vi "nanocal -- nuclear schottky fit -- 2x2 -- V9.vi"() -> ()   [LabVIEW 2021] (continued)
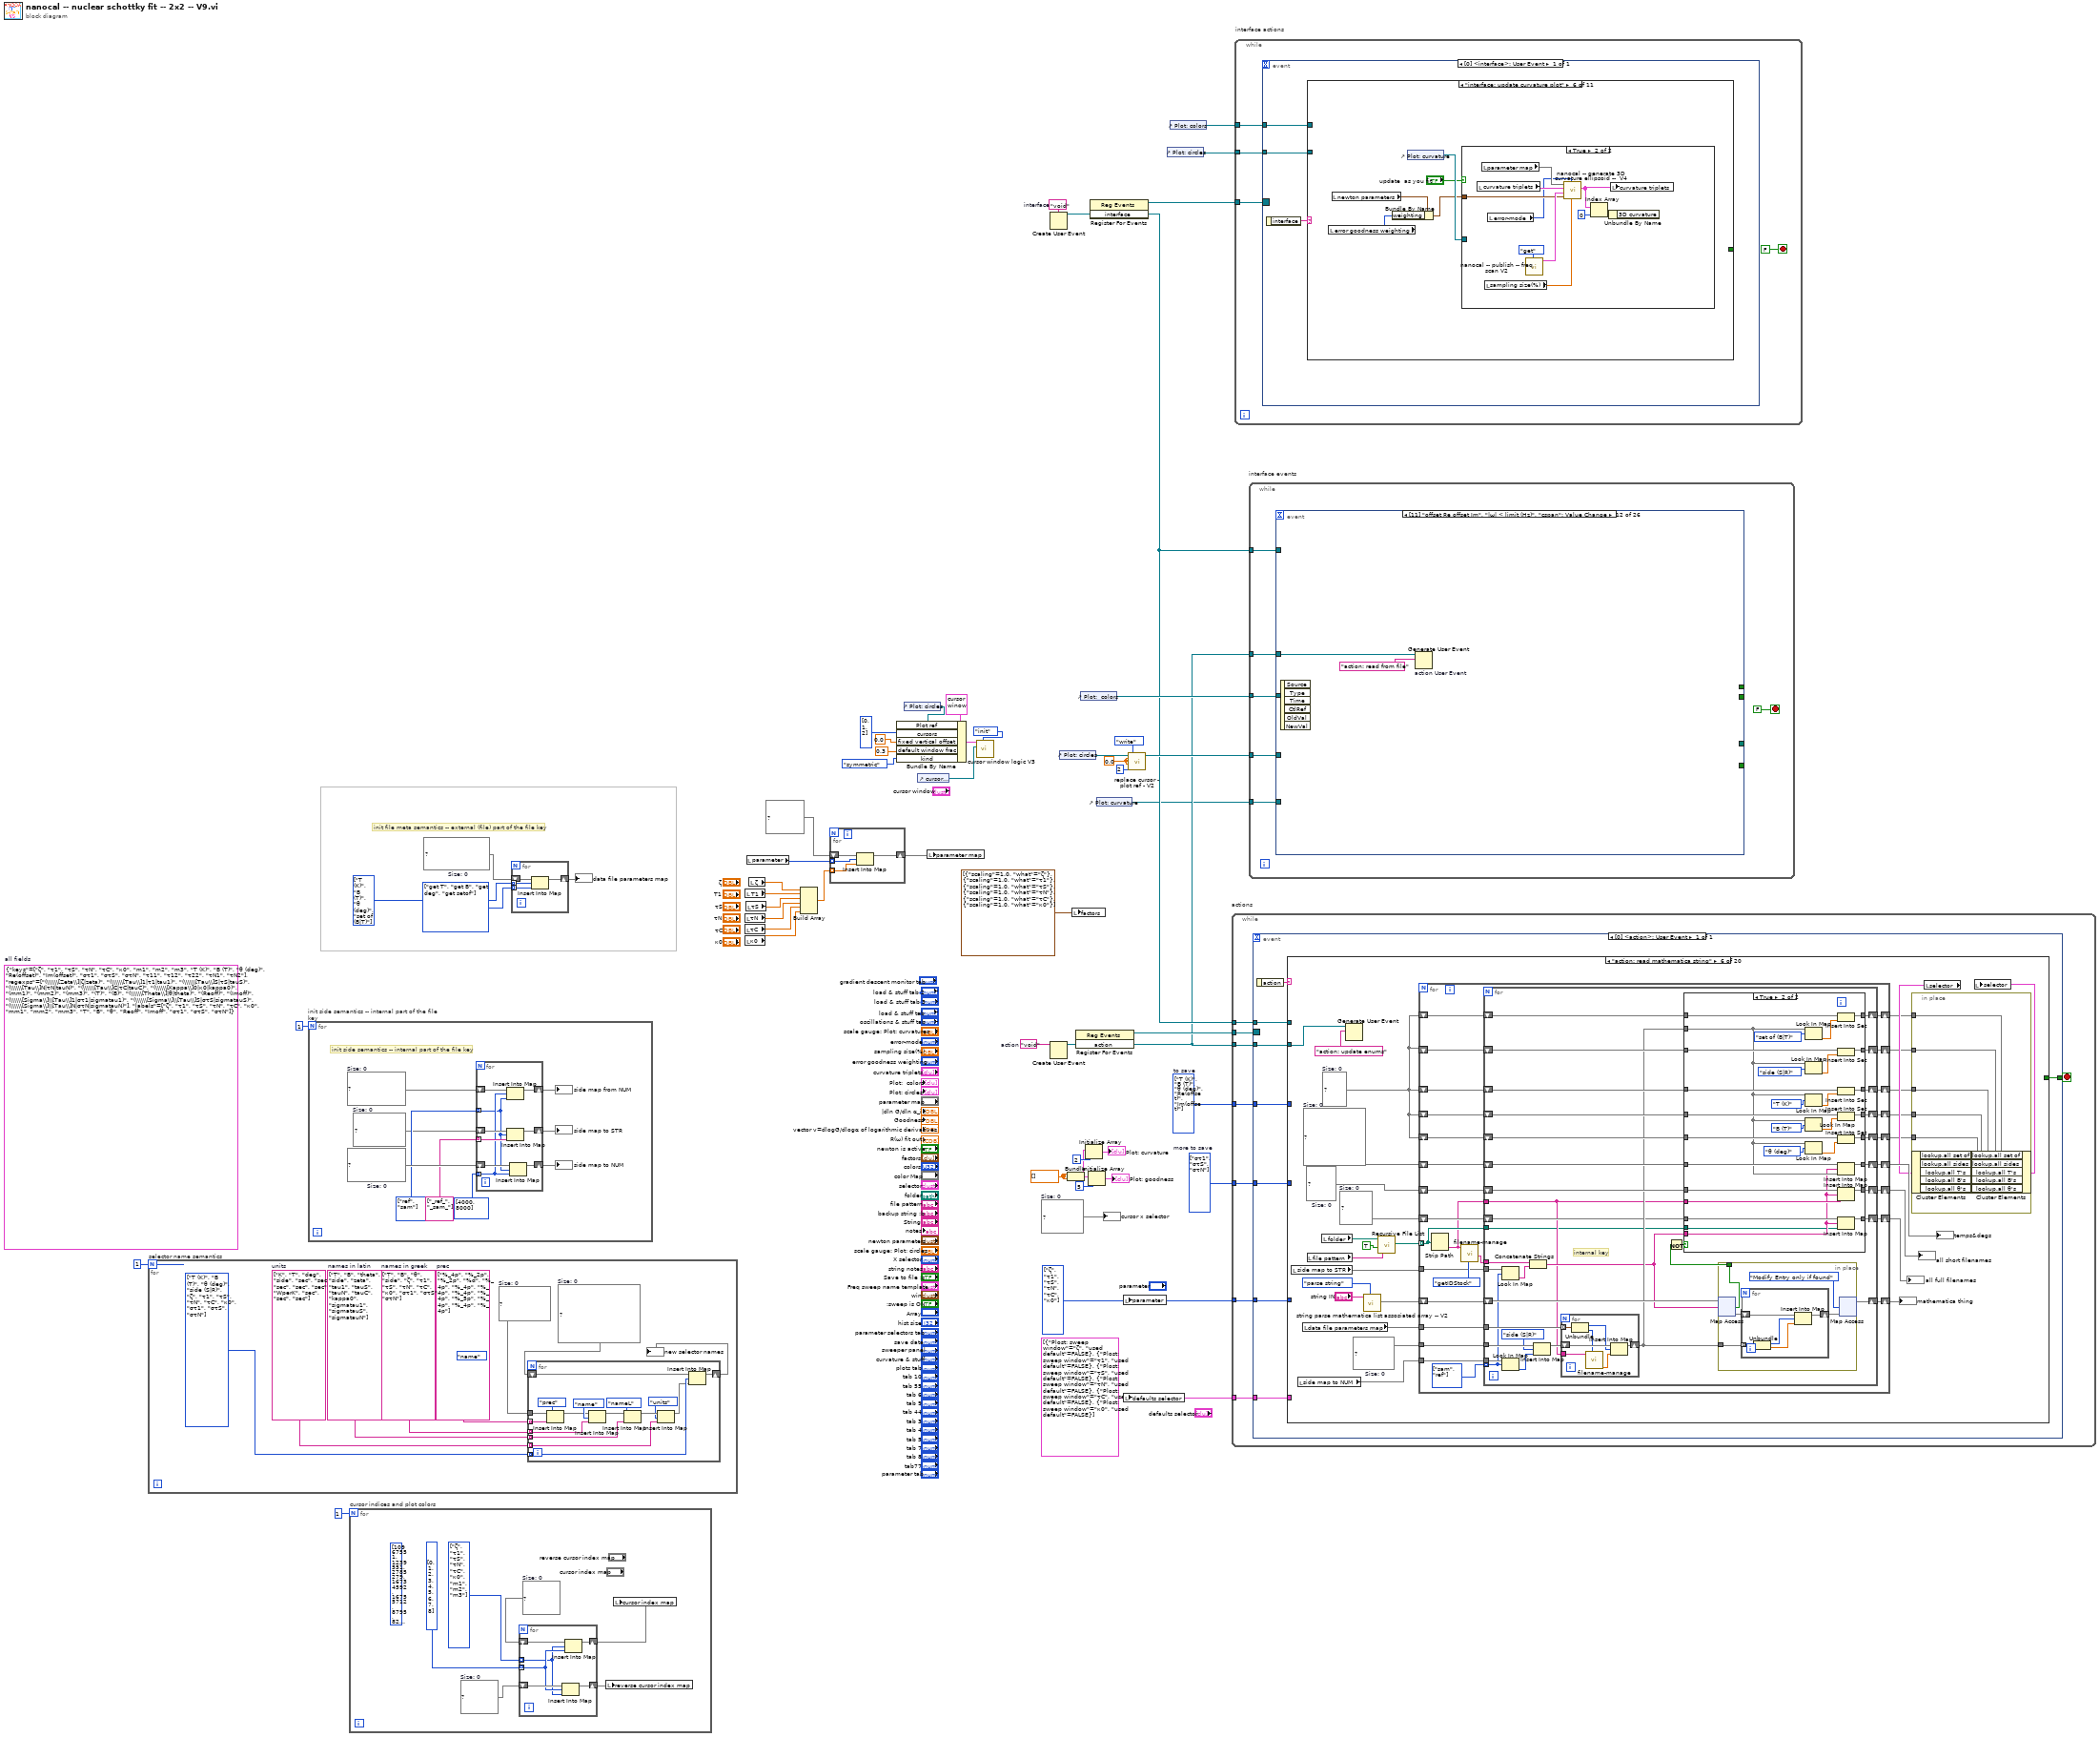
[diagram p0: block diagram]
diagram:
  w1 = T2[] [enum."T (K)", enum."B (T)", enum."θ (deg)", enum."Re(offset)", enum."Im(offset)"] items=["ζ", "τ1", "τS", "τN", "τC", "κ0", "m1", "m2", "m3", "T (K)", "B (T)", "θ (deg)", "side (S|R)", "set of (B|T)", "Re(offset)", "Im(offset)", "στ1", "στ1-", "στ1+", "στS", "στS-", "στS+", "στN", "στN-", "στN+", "τ11", "τ12", "τ21", "τ22", "τN1", "τN2"]  # to save
  w2 = T2[] [enum."στ1", enum."στS", enum."στN"] items=["ζ", "τ1", "τS", "τN", "τC", "κ0", "m1", "m2", "m3", "T (K)", "B (T)", "θ (deg)", "side (S|R)", "set of (B|T)", "Re(offset)", "Im(offset)", "στ1", "στ1-", "στ1+", "στS", "στS-", "στS+", "στN", "στN-", "στN+", "τ11", "τ12", "τ21", "τ22", "τN1", "τN2"]  # more to save
  (unwired) T20 {"keys"=[enum."ζ", enum."τ1", enum."τS", enum."τN", enum."τC", enum."κ0", enum."m1", enum."m2", enum."m3", enum."T (K)", enum."B (T)", enum."θ (deg)", enum."Re(offset)", enum."Im(offset)", enum."στ1", enum."στS", enum."στN", enum."τ11", enum."τ12", enum."τ22", enum."τN1", enum."τN2"], "regexps"=["(\\\\\\[Zeta\\]|ζ|zeta)", "(\\\\\\[Tau\\]1|τ1|tau1)", "(\\\\\\[Tau\\]S|τS|tauS)", "(\\\\\\[Tau\\]N|τN|tauN)", "(\\\\\\[Tau\\]C|τC|tauC)", "(\\\\\\[Kappa\\]0|κ0|kappa0)", "(mm1)", "(mm2)", "(mm3)", "(T)", "(B)", "(\\\\\\[Theta\\]|θ|theta)", "(Reoff)", "(Imoff)", "(\\\\\\[Sigma\\]\\[Tau\\]1|στ1|sigmatau1)", "(\\\\\\[Sigma\\]\\[Tau\\]S|στS|sigmatauS)", "(\\\\\\[Sigma\\]\\[Tau\\]N|στN|sigmatauN)"], "labels"=["ζ", "τ1", "τS", "τN", "τC", "κ0", "mm1", "mm2", "mm3", "T", "B", "θ", "Reoff", "Imoff", "στ1", "στS", "στN"]}  # all fields
  w26 = T9 [{"Plost: sweep window"=enum."ζ", "used default"=FALSE}, {"Plost: sweep window"=enum."τ1", "used default"=FALSE}, {"Plost: sweep window"=enum."τS", "used default"=FALSE}, {"Plost: sweep window"=enum."τN", "used default"=FALSE}, {"Plost: sweep window"=enum."τC", "used default"=FALSE}, {"Plost: sweep window"=enum."κ0", "used default"=FALSE}] ("parameter 2")
  w27 = T18[] [enum."get T", enum."get B", enum."get deg", enum."get setof"] items=["rewrite", "parse", "force pattern", "uniquenum", "get T", "get B", "get ind", "get deg", "get name", "get folder", "get extension", "get basename", "get side", "get setof", "getID", "getIDStock"]
  w29 = map{T2, T18} {}  # Size: 0
  w28 = T2[] [enum."T (K)", enum."B (T)", enum."θ (deg)", enum."set of (B|T)"] items=["ζ", "τ1", "τS", "τN", "τC", "κ0", "m1", "m2", "m3", "T (K)", "B (T)", "θ (deg)", "side (S|R)", "set of (B|T)", "Re(offset)", "Im(offset)", "στ1", "στ1-", "στ1+", "στS", "στS-", "στS+", "στN", "στN-", "στN+", "τ11", "τ12", "τ21", "τ22", "τN1", "τN2"]
  w33 = dbl[] []
  w22 = T2[] [enum."ζ", enum."τ1", enum."τS", enum."τN", enum."τC", enum."κ0"] items=["ζ", "τ1", "τS", "τN", "τC", "κ0", "m1", "m2", "m3", "T (K)", "B (T)", "θ (deg)", "side (S|R)", "set of (B|T)", "Re(offset)", "Im(offset)", "στ1", "στ1-", "στ1+", "στS", "στS-", "στS+", "στN", "στN-", "στN+", "τ11", "τ12", "τ21", "τ22", "τN1", "τN2"]
  w36 = map{T2, dbl} {}  # Size: 0
  w37 = 0.0 ("new X")
  w50 = "void"  # interface
  w51 = "void"  # action
  # "init file meta semantics -- external (file) part of the file key"
  n1 = for "selector name semantics" {
    N: 1 -> [_]
    w53 = string[] ["%_4p", "%_2p", "%_2p", "%d", "%_4p", "%_4p", "%_4p", "%_4p", "%_4p", "%_5p", "%_4p", "%_4p", "%_4p"]  # prec
    w57 = map{T19, string} {}  # Size: 0
    (unwired) nameformattingitem."name" ("name formatting item")
    w55 = string[] ["K", "T", "deg", "side", "sec", "sec", "sec", "sec", "sec", "WperK", "sec", "sec", "sec"]  # units
    w58 = string[] ["T", "B", "theta", "side", "zeta", "tau1", "tauS", "tauN", "tauC", "kappa0", "sigmatau1", "sigmatauS", "sigmatauN"]  # names in latin
    w56 = string[] ["T", "B", "θ", "side", "ζ", "τ1", "τS", "τN", "τC", "κ0", "στ1", "στS", "στN"]  # names in greek
    w60 = map{T2, map{T19, string}} {}  # Size: 0
    w59 = T2[] [enum."T (K)", enum."B (T)", enum."θ (deg)", enum."side (S|R)", enum."ζ", enum."τ1", enum."τS", enum."τN", enum."τC", enum."κ0", enum."στ1", enum."στS", enum."στN"] items=["ζ", "τ1", "τS", "τN", "τC", "κ0", "m1", "m2", "m3", "T (K)", "B (T)", "θ (deg)", "side (S|R)", "set of (B|T)", "Re(offset)", "Im(offset)", "στ1", "στ1-", "στ1+", "στS", "στS-", "στS+", "στN", "στN-", "στN+", "τ11", "τ12", "τ21", "τ22", "τN1", "τN2"]
    n2 = for {
      shift-right: [w75] -> w54
      shift-left: w60 -> [w76]
      tunnel: w58 -> [w66] mode=indexing
      tunnel: w59 -> [w74] mode=indexing
      tunnel: w57 -> [w64]
      tunnel: w56 -> [w65] mode=indexing
      tunnel: w55 -> [w67] mode=indexing
      tunnel: w53 -> [w63] mode=indexing
      n3 = Insert Into Map(map in=w64, key=nameformattingitem."prec", value=w63) -> (map out=w62:map{T19, string})  [unwired: 2 out]
      n4 = Insert Into Map(map in=w62, key=nameformattingitem."name", value=w65) -> (map out=w73:map{T19, string})  [unwired: 2 out]
      n5 = Insert Into Map(map in=w73, key=nameformattingitem."nameL" ("name formatting item"), value=w66) -> (map out=w72:map{T19, string})  [unwired: 2 out]
      n6 = Insert Into Map(map in=w72, key=nameformattingitem."units" ("name formatting item"), value=w67) -> (map out=w71:map{T19, string})  [unwired: 2 out]
      n7 = Insert Into Map(map in=w76, key=w74, value=w71) -> (map out=w75:map{T2, map{T19, string}})  [unwired: 2 out]
    }
    "new selector names" <- w54
  }
  n8 = for "init side semantics -- internal part of the file key" {
    N: 1 -> [_]
    w78 = map{i32, T8} {}  # Size: 0
    w80 = map{T8, string} {}  # Size: 0
    w81 = T8[] [enum."ref", enum."sam"] items=["sam", "ref"]
    w85 = map{T8, i32} {}  # Size: 0
    # "init side semantics -- internal part of the file key"
    n9 = for {
      shift-right: [w93] -> w82
      shift-left: w85 -> [w94]
      tunnel: string[] ["_ref_", "_sam_"] -> [w90] mode=indexing
      tunnel: i32[] [4000, 8000] -> [w87] mode=indexing
      tunnel: w81 -> [w86] mode=indexing
      shift-right: [w91] -> w79
      shift-left: w80 -> [w92]
      shift-right: [w88] -> w77
      shift-left: w78 -> [w89]
      n10 = Insert Into Map(map in=w89, key=w87, value=w86) -> (map out=w88:map{i32, T8})  [unwired: 2 out]
      n11 = Insert Into Map(map in=w92, key=w86, value=w90) -> (map out=w91:map{T8, string})  [unwired: 2 out]
      n12 = Insert Into Map(map in=w94, key=w86, value=w87) -> (map out=w93:map{T8, i32})  [unwired: 2 out]
    }
    "side map from NUM" <- w77
    "side map to STR" <- w79
    "side map to NUM" <- w82
  }
  n13 = for "cursor indices and plot colors" {
    N: 1 -> [_]
    w96 = map{i32, T2} {}  # Size: 0
    (unwired) u32[] [10967551, 1239551, 2785279, 16734592, 16755712, 8795, 8285330, 9272482, 9204890]
    w100 = map{T2, i32} {}  # Size: 0
    w97 = T2[] [enum."ζ", enum."τ1", enum."τS", enum."τN", enum."τC", enum."κ0", enum."m1", enum."m2", enum."m3"] items=["ζ", "τ1", "τS", "τN", "τC", "κ0", "m1", "m2", "m3", "T (K)", "B (T)", "θ (deg)", "side (S|R)", "set of (B|T)", "Re(offset)", "Im(offset)", "στ1", "στ1-", "στ1+", "στS", "στS-", "στS+", "στN", "στN-", "στN+", "τ11", "τ12", "τ21", "τ22", "τN1", "τN2"]
    n14 = for {
      shift-right: [w105] -> w98
      shift-left: w100 -> [w106]
      tunnel: w97 -> [w101] mode=indexing
      tunnel: i32[] [0, 1, 2, 3, 4, 5, 6, 7, 8] -> [w102] mode=indexing
      shift-right: [w103] -> w95
      shift-left: w96 -> [w104]
      n15 = Insert Into Map(map in=w104, key=w102, value=w101) -> (map out=w103:map{i32, T2})  [unwired: 2 out]
      n16 = Insert Into Map(map in=w106, key=w101, value=w102) -> (map out=w105:map{T2, i32})  [unwired: 2 out]
    }
    n17 = local write "reverse cursor index map"(w95) -> ()
    n18 = local write "cursor index map"(w98) -> ()
  }
  n19 = for {
    shift-right: [w109] -> w30
    shift-left: w29 -> [w110]
    tunnel: w28 -> [w108] mode=indexing
    tunnel: w27 -> [w107] mode=indexing
    n20 = Insert Into Map(map in=w110, key=w108, value=w107) -> (map out=w109:map{T2, T18})  [unwired: 2 out]
  }
  "data file parameters map" <- w30
  n21 = local read "τN"() -> (w16:dbl)
  n22 = local read "τC"() -> (w17:dbl)
  n23 = local read "κ0"() -> (w18:dbl)
  n24 = local read "T1"() -> (w14:dbl)
  n25 = local read "τS"() -> (w15:dbl)
  n26 = local read "parameter"() -> (w20:T2[])
  n27 = local read "ζ"() -> (w13:dbl)
  n28 = Build Array(w13, w14, w15, w16, w17, w18) -> (w19:dbl[])
  n29 = for {
    shift-right: [w113] -> w21
    shift-left: map{T2, dbl} {} ("Map IN") -> [w114]
    tunnel: w20 -> [w112] mode=indexing
    tunnel: w19 -> [w111] mode=indexing
    n30 = Insert Into Map(map in=w114, key=w112, value=w111) -> (map out=w113:map{T2, dbl})  [unwired: 2 out]
  }
  n31 = control-ref of="Plot: circles"() -> (w42:refnum<vi>)
  n32 = Bundle By Name(cluster=T17 {"left"=0.0, "right "=0.0, "center"=0.0, "window"=0.0, "cursors"=[], "relative"=0, "absolute"=0, "fixed vertical offset"=0.0, "vertical offset"=0.0, "skew"=0.0, "default window frac"=0.0, "kind"=enum."symmetric", "skew.left"=0.0, "skew.right"=0.0, "Plot ref"=refnum, "wing order"=enum."forw"} ("cursor bracket: All, data window"), "Plot ref"=w42, "cursors"=i32[] [0, 1, 2], "fixed vertical offset"=0.0, "default window frac"=0.3 ("fixed vertical offset"), "kind"=enum16{"symmetric", "skewed", "fancy"}."symmetric") -> (w45:T17)
  n33 = control-ref of="cursor window"() -> (w41:refnum<vi>)
  n34 = local write "parameter map"(w21) -> ()
  n35 = call "cursor window logic V3.vi"("cursor window action"=cursor_window_action."init", "cursor window in"=w41, "cursor window init"=w45) -> ()  [unwired: 7 in, 2 out]
  n36 = Create User Event(user event datatype=w50) -> (user event=w10:refnum<user-event>)  [unwired: 1 in, 1 out]
  n37 = Create User Event(user event datatype=w51) -> (user event=w9:refnum<user-event>)  [unwired: 1 in, 1 out]
  n38 = control-ref of="Plot: circles"() -> (w38:refnum<vi>)
  n39 = Bundle(w33, w33) -> (w5:cluster{dbl[], dbl[]})  [unwired: 1 in]
  n40 = local write "factors"(cluster{"scaling":dbl, "what":T2}[] [{"scaling"=1.0, "what"=enum."ζ"}, {"scaling"=1.0, "what"=enum."τ1"}, {"scaling"=1.0, "what"=enum."τS"}, {"scaling"=1.0, "what"=enum."τN"}, {"scaling"=1.0, "what"=enum."τC"}, {"scaling"=1.0, "what"=enum."κ0"}]) -> ()
  n41 = register-events(w9) -> (reference out=w52:refnum<event-registration>)  [unwired: 2 in, 1 out]
  n42 = control-ref of="Plot:  colors"() -> (w35:refnum<vi>)
  n43 = Initialize Array(w5, 2 ("dimension size")) -> (→"Plot: curvature":cluster{dbl[], dbl[]}[])
  n44 = Initialize Array(w5, 5 ("dimension size")) -> (→"Plot: goodness":cluster{dbl[], dbl[]}[])
  n45 = register-events(w10) -> (reference out=w11:refnum<event-registration>)  [unwired: 2 in, 1 out]
  n46 = control-ref of="Plot: curvature"() -> (w3:refnum<vi>)
  n47 = local write "parameter"(w22) -> ()
  n48 = local write "defaults selector"(w26) -> ()
  n49 = call "replace cursor - plot ref - V2.vi"("Plot ref in"=w38, "new X"=w37, "new  Y"=w37, "cursor index"=2, "cursor action"=cursor_action."write") -> ()  [unwired: 11 in, 4 out]
  n50 = control-ref of="Plot: circles"() -> (w7:refnum<vi>)
  n51 = control-ref of="Plot: colors"() -> (w8:refnum<vi>)
  n52 = while "actions" {
    tunnel: w52 -> [w122]
    tunnel: w9 -> [w121]
    tunnel: w10 -> [w119]
    tunnel: w22 -> [w118]
    tunnel: w26 -> [w117]
    tunnel: w2 -> [w116]
    tunnel: w1 -> [w115]
    stop <- w120 stop-if-true
    n53 = event shown="[0] <action>: User Event" {
      selector: w122 -> [_]
      dyn-events: _ -> [_]
      timeout: _ -> [_]
      tunnel: w121 -> [w129]
      tunnel: [w128] -> w120
      tunnel: w119 -> [w127]
      tunnel: w118 -> [w126]
      tunnel: w117 -> [w125]
      tunnel: w116 -> [w124]
      tunnel: w115 -> [w123]
      event User Event {
        n54 = event-data() -> ("action"=w130:string)  [unwired: 1 in]
        n55 = case shown="\"action: read mathematica string\"" w130 {
          tunnel: w129 -> [w138 _ _ _ w321 w346 _ _ w539 _ w666 _ _ w772 w824 w925 _ w987 _ _]
          tunnel: [_ _ _ _ _ _ _ _ _ _ _ _ _ _ _ _ TRUE _ _ _] -> w128
          tunnel: w127 -> [w141 w145 _ w266 w315 _ _ _ _ _ _ _ w682 _ w814 _ _ _ _ _]
          tunnel: w126 -> [_ w152 w161 w265 _ _ w473 _ _ _ _ _ w680 _ w820 _ _ _ _ _]
          tunnel: w125 -> [_ _ _ _ _ _ _ _ _ _ _ _ _ _ _ _ _ _ _ _]
          tunnel: w124 -> [_ _ _ _ _ _ _ _ _ _ _ _ w678 _ _ w896 _ _ _ _]
          tunnel: w123 -> [_ _ _ _ _ _ _ _ _ _ _ _ _ _ _ w893 _ _ _ _]
          frame "action: new sweep" {
            n56 = Generate User Event(user event=w141, event data cluster="interface: update plot colors cursors" ("event data")) -> (user event out=w142:refnum<user-event>)  [unwired: 2 in, 1 out]
            n57 = Generate User Event(user event=w142, event data cluster="interface: reset colors" ("event data")) -> ()  [unwired: 2 in, 2 out]
            n58 = Generate User Event(user event=w138, event data cluster="action: replot circles" ("event data")) -> ()  [unwired: 2 in, 2 out]
            n59 = call "nanocal -- publish -- freq scan V2.vi"("publisher action"=publisher_action."get") -> ("z out (V)"=w137:cdb[])  [unwired: 7 in, 3 out]
            n60 = control-ref of="Plot: circles"() -> (w132:refnum<vi>)
            n61 = Complex To Re/Im(x + iy=w137) -> (x=w135:dbl[], y=w136:dbl[])
            n62 = call "replace plot - plot ref - V2.vi"("Plot ref in"=w132, "Array X IN"=w135, "Array Y IN"=w136, "plot index"=enum16{"data R(ω)", "fit R(ω)"}."data R(ω)" ("Plost: sweep window"), "cursor action"=cursor_action."write") -> ()  [unwired: 11 in, 4 out]
          }
          frame "action: replot circles" {
            n63 = local read "newton parameters"() -> (w153:T3)
            n64 = local read "parameter map"() -> (w147:map{T2, dbl})
            n65 = call "nanocal -- publish -- freq scan V2.vi"("publisher action"=publisher_action."get") -> ("data"=w151:T34)  [unwired: 7 in, 3 out]
            n66 = call "nanocal -- gradient descent.vi"("data"=w151, "action"=nanocal_--_gradient_descent_--_action."peek", "newton pars"=w153, "parameter keys IN"=w152, "parameter Map IN"=w147) -> ("logarithmic derivatives OUT"=w148:dbl[], "R(ω) out"=w146:cdb[], "goodness OUT"=w150:dbl)  [unwired: 2 in, 2 out]
            n67 = local write "vector v=dlogG/dlogα of logarithmic derivatives"(w148) -> ()
            n68 = Absolute Value(x=w148) -> (abs(x)=w149:dbl[])
            n69 = flat-sequence {
              tunnel: w146 -> [w156]
              tunnel: w145 -> [w158]
              tunnel: "interface: update circle fit plot" ("event data") -> [w157]
              frame #0 {
                n70 = local write "R(ω) fit out"(w156) -> ()
              }
              frame #1 {
                n71 = Generate User Event(user event=w158, event data cluster=w157) -> ()  [unwired: 2 in, 2 out]
              }
            }
            n72 = local write "Goodness"(w150) -> ()
            n73 = local write "|v_i| = | dlogG/dlogα_i | (log scale slider)"(w149) -> ()
          }
          frame "action: plot landscape" {
            w172 = array_action."generate log range" ("action")
            n74 = property on="range one" class="Slide (strict)"() -> ("Scale.Range"=w181:T36)  [unwired: 2 in, 2 out]
            n75 = property on="range two" class="Slide (strict)"() -> ("Scale.Range"=w180:T36)  [unwired: 2 in, 2 out]
            n76 = Unbundle By Name(w181) -> ("Maximum"=w175:dbl, "Minimum"=w174:dbl)
            n77 = Unbundle By Name(w180) -> ("Maximum"=w177:dbl, "Minimum"=w176:dbl)
            n78 = local read "cursor index map"() -> (w167:map{T2, i32})
            n79 = call "array -- generate range -- V5.vi"("action"=w172, "ω points"="# points", "ω from"=w176, "ω to"=w177) -> ("ω out"=w178:dbl[])  [unwired: 7 in]
            n80 = local read "color Map"() -> (w168:map{T2, u32})
            n81 = call "array -- generate range -- V5.vi"("action"=w172, "ω points"="# points", "ω from"=w174, "ω to"=w175) -> ("ω out"=w173:dbl[])  [unwired: 7 in]
            n82 = call "nanocal -- publish -- freq scan V2.vi"("publisher action"=publisher_action."get") -> ("data"=w160:T34)  [unwired: 7 in, 3 out]
            n83 = local read "newton parameters"() -> (w162:T3)
            n84 = local read "parameter map"() -> (w159:map{T2, dbl})
            n85 = Look In Map(map=w168, key="two") -> (value=w170:u32)  [unwired: 1 in, 1 out]
            n86 = Look In Map(map=w168, key="one") -> (value=w169:u32)  [unwired: 1 in, 1 out]
            n87 = Build Array("one", "two") -> (w166:T2[])
            n88 = property on="range one" class="Slide (strict)"("Fill Color"=w169) -> ()  [unwired: 2 in, 2 out]
            n89 = property on="range two" class="Slide (strict)"("Fill Color"=w170) -> ()  [unwired: 2 in, 2 out]
            n90 = case shown="\"1d plots\", Default" "what" {
              tunnel: w159 -> [w189 w229]
              tunnel: "one" -> [_ w228]
              tunnel: w178 -> [_ w227]
              tunnel: w173 -> [w188 w226]
              tunnel: "two" -> [_ w225]
              tunnel: w168 -> [w187 _]
              tunnel: w167 -> [w186 _]
              tunnel: w166 -> [w183 _]
              tunnel: w160 -> [w184 w220]
              tunnel: w162 -> [w182 w218]
              tunnel: w161 -> [_ w219]
              frame "1d plots", Default {
                n91 = control-ref of="Plot: goodness"() -> (w185:refnum<vi>)
                n92 = for {
                  tunnel: w189 -> [w196]
                  tunnel: w188 -> [w205]
                  tunnel: w183 -> [w195] mode=indexing
                  tunnel: w187 -> [w202]
                  tunnel: w186 -> [w201]
                  tunnel: w185 -> [w193]
                  tunnel: w184 -> [w192]
                  tunnel: w183 -> [w191]
                  tunnel: w182 -> [w190]
                  n93 = for {
                    tunnel: w205 -> [w209] mode=indexing
                    tunnel: [w210] -> w207 mode=indexing
                    tunnel: [w209] -> w206 mode=indexing
                    tunnel: w196 -> [w216]
                    tunnel: w195 -> [w217]
                    tunnel: w192 -> [w215]
                    tunnel: w191 -> [w212]
                    tunnel: w190 -> [w211]
                    n94 = Insert Into Map(map in=w216, key=w217, value=w209) -> (map out=w214:map{T2, dbl})  [unwired: 2 out]
                    n95 = call "nanocal -- gradient descent.vi"("data"=w215, "action"=nanocal_--_gradient_descent_--_action."peek", "newton pars"=w211, "parameter keys IN"=w212, "parameter Map IN"=w214) -> ("goodness OUT"=w210:dbl)  [unwired: 2 in, 4 out]
                  }
                  n96 = Look In Map(map=w196, key=w195) -> (value=w194:dbl)  [unwired: 1 in, 1 out]
                  n97 = Look In Map(map=w202, key=w195) -> (value=w197:u32)  [unwired: 1 in, 1 out]
                  n98 = Look In Map(map=w201, key=w195) -> (value=w199:i32)  [unwired: 1 in, 1 out]
                  n99 = call "replace plot - plot ref - V2.vi"("Plot ref in"=w193, "Array X IN"=w206, "Array Y IN"=w207, "plot index"=w199, "cursor action"=cursor_action."write") -> ("Plot ref out"=w204:refnum<vi>)  [unwired: 11 in, 3 out]
                  n100 = call "replace cursor - plot ref - V2.vi"("Plot ref in"=w193, "new X"=w194, "cursor index"=w199, "cursor action"=cursor_action."write", "Color Box"=w197, "cursor state"=cursor_sate."colored") -> ()  [unwired: 10 in, 4 out]
                  n101 = call "replace plot - plot ref - V2.vi"("Plot ref in"=w204, "plot index"=w199, "cursor action"=cursor_action."set plot color", "Color Box"=w197) -> ()  [unwired: 12 in, 4 out]
                }
              }
              frame "2d plots " {
                n102 = for {
                  tunnel: w229 -> [w239]
                  tunnel: w228 -> [w238]
                  tunnel: w227 -> [w237] mode=indexing
                  tunnel: w226 -> [w236]
                  tunnel: w225 -> [w235]
                  shift-right: [w233] -> w222
                  shift-left: "{ " -> [w234]
                  tunnel: w220 -> [w232]
                  tunnel: w219 -> [w231]
                  tunnel: w218 -> [w230]
                  n103 = for {
                    tunnel: w236 -> [w247] mode=indexing
                    tunnel: w237 -> [w246]
                    tunnel: w239 -> [w260]
                    tunnel: w238 -> [w261]
                    tunnel: w235 -> [w259]
                    shift-right: [w256] -> w233
                    shift-left: w234 -> [w257]
                    tunnel: w232 -> [w244]
                    tunnel: w231 -> [w241]
                    tunnel: w230 -> [w240]
                    w250 = " ,     "
                    w255 = i16 12 ("precision (6)")
                    n104 = Insert Into Map(map in=w260, key=w261, value=w247) -> (map out=w258:map{T2, dbl})  [unwired: 2 out]
                    n105 = Number To Fractional String(number=w247, precision (6)=w255) -> (F-format string=w254:string)  [unwired: 2 in]
                    n106 = Number To Fractional String(number=w246, precision (6)=w255) -> (F-format string=w253:string)  [unwired: 2 in]
                    n107 = Insert Into Map(map in=w258, key=w259, value=w246) -> (map out=w245:map{T2, dbl})  [unwired: 2 out]
                    n108 = call "nanocal -- gradient descent.vi"("data"=w244, "action"=nanocal_--_gradient_descent_--_action."peek", "newton pars"=w240, "parameter keys IN"=w241, "parameter Map IN"=w245) -> ("goodness OUT"=w242:dbl)  [unwired: 2 in, 4 out]
                    n109 = Number To Fractional String(number=w242, precision (6)=w255) -> (F-format string=w252:string)  [unwired: 2 in]
                    n110 = Concatenate Strings(w257, "{    ", w254, w250, w253, w250, w252, " } , ", "\r") -> (w256:string)
                  }
                }
                n111 = Concatenate Strings(w222, " }   ") -> (→"2dplots":string)
              }
            }
          }
          frame "action: gradient step" {
            n112 = local write "newton is active"(TRUE ("newton is active")) -> ()
            n113 = call "nanocal -- publish -- freq scan V2.vi"("publisher action"=publisher_action."get") -> ("data"=w267:T34)  [unwired: 7 in, 3 out]
            n114 = call "nanocal -- gradient descent.vi"("data"=w267, "action"=nanocal_--_gradient_descent_--_action."init") -> ("goodness OUT"=w269:dbl)  [unwired: 5 in, 4 out]
            n115 = while {
              tunnel: w269 -> [_]
              tunnel: w265 -> [w289]
              tunnel: w266 -> [w279]
              tunnel: [w274] -> w263
              i -> [w275]
              stop <- w274 continue-if-true
              n116 = local read "newton is active"() -> (w290:bool)
              n117 = local read "factors"() -> (w293:cluster{"scaling":dbl, "what":T2}[])
              n118 = local read "newton parameters"() -> (w288:T3)
              n119 = Quotient & Remainder(x=w275, y="update rate") -> (x-y*floor(x/y)=w278:i32)  [unwired: 1 out]
              n120 = Less?(x=w275, y="total # steps") -> (x < y?=w276:bool)
              n121 = for {
                shift-right: [w313] -> w282
                shift-left: map{T2, dbl} {} ("Map IN") -> [w314]
                tunnel: w293 -> [w312] mode=indexing
                n122 = Unbundle(w312) -> ("scaling"=w310:dbl, "what"=w311:T2)
                n123 = Insert Into Map(map in=w314, key=w311, value=w310) -> (map out=w313:map{T2, dbl})  [unwired: 2 out]
              }
              n124 = local read "parameter map"() -> (w283:map{T2, dbl})
              n125 = And(x=w276, y=w290) -> (x .and. y?=w274:bool)
              n126 = case shown="0" w278 {
                tunnel: w279 -> [_ w297]
                frame 1, Default {
                }
                frame 0 {
                  n127 = Generate User Event(user event=w297, event data cluster="interface: update list from parameter map" ("event data")) -> (user event out=w296:refnum<user-event>)  [unwired: 2 in, 1 out]
                  n128 = Generate User Event(user event=w296, event data cluster="interface: update plot colors cursors" ("event data")) -> (user event out=w300:refnum<user-event>)  [unwired: 2 in, 1 out]
                  n129 = Generate User Event(user event=w300, event data cluster="interface: update circle fit plot" ("event data")) -> (user event out=w295:refnum<user-event>)  [unwired: 2 in, 1 out]
                  n130 = Generate User Event(user event=w295, event data cluster="interface: update curvature plot" ("event data")) -> ()  [unwired: 2 in, 2 out]
                }
              }
              n131 = call "nanocal -- gradient descent.vi"("# steps"="#grad steps", "action"=nanocal_--_gradient_descent_--_action."step", "newton pars"=w288, "parameter keys IN"=w289, "parameter Map IN"=w283, "factors Map IN"=w282) -> ("logarithmic derivatives OUT"=w284:dbl[], "step factors OUT"=w291:map{T2, dbl}, "R(ω) out"=w281:cdb[], "goodness OUT"=w271:dbl, "oscillations"=→"Plot: oscillations":cluster{"Array":i32[], "Array":dbl[]})  [unwired: 1 in]
              n132 = for {
                tunnel: w289 -> [w302] mode=indexing
                shift-right: [w306] -> _
                shift-left: w291 -> [w306]
                shift-right: [w304] -> w272
                shift-left: w283 -> [w305]
                n133 = Look In Map(map=w306, key=w302) -> (value=w303:dbl)  [unwired: 1 in, 1 out]
                n134 = in-place {
                  in-place-border: w303 -> [w308]
                  n135 = in-place-map #1(w305, w302) -> (w309:dbl)  [unwired: 1 in, 1 out]
                  n136 = Multiply(x=w308, y=w309) -> (x*y=w307:dbl)
                  n137 = in-place-map #1(w307) -> (w304:map{T2, dbl})  [unwired: 1 in, 2 out]
                }
              }
              n138 = Absolute Value(x=w284) -> (abs(x)=→"|v_i| = | dlogG/dlogα_i | (log scale slider)":dbl[])
              n139 = local write "vector v=dlogG/dlogα of logarithmic derivatives"(w284) -> ()
              n140 = local write "R(ω) fit out"(w281) -> ()
              n141 = local write "Goodness"(w271) -> ()
              n142 = local write "parameter map"(w272) -> ()
              "current step ind" <- w275
            }
            n143 = local write "newton is active"(w263) -> ()
            "current  ind" <- 0 ("plot ind")
          }
          frame "action: parse string" {
            n144 = local read "String"() -> (w323:string)
            n145 = Generate User Event(user event=w315, event data cluster="interface: update list from parameter map" ("event data")) -> ()  [unwired: 2 in, 2 out]
            n146 = call "string parse mathematica assosiated array.vi"("action"=mathematica_string_map_action."parse string" ("derivative"), "String in"=w323) -> ("Map OUT"=w317:map{T2, dbl})  [unwired: 8 in, 1 out]
            n147 = Generate User Event ("action User Event")(user event=w321, event data cluster="action: update state of selectors" ("event data")) -> (user event out=w318:refnum<user-event>)  [unwired: 2 in, 1 out]
            n148 = Generate User Event ("action User Event")(user event=w318, event data cluster="action: replot colors" ("event data")) -> ()  [unwired: 2 in, 2 out]
            n149 = local write "parameter map"(w317) -> ()
          }
          frame "action: read mathematica string" {
            w333 = map{string, path} {}  # Size: 0
            w348 = map{T2, dbl} {}  # Size: 0
            w345 = set{dbl} {}  # Size: 0
            w349 = map{string, map{T2, dbl}} {}  # Size: 0
            w339 = map{string, string} {}  # Size: 0
            n150 = local read "side map to STR"() -> (w341:map{T8, string})
            n151 = local read "side map to NUM"() -> (w340:map{T8, i32})
            n152 = local read "data file parameters map"() -> (w342:map{T2, T18})
            n153 = local read "file pattern"() -> (w336:string)
            n154 = local read "folder"() -> (w337:path)
            n155 = Generate User Event(user event=w346, event data cluster="action: update enums" ("event data")) -> ()  [unwired: 2 in, 2 out]
            n156 = call "string parse mathematica list assosiated array -- V2.vi"("action"=3-lorentzian-heat-response_action."parse string" ("derivative"), "string IN"="string IN") -> ("Map OUT"=w350:map{string, map{T2, dbl}})  [unwired: 8 in, 1 out]
            n157 = call <vilib>:"Recursive File List.vi"("pattern"=w336, "Continue Recursing on Error? (F)"=TRUE, "Folder Path"=w337) -> ("All Files in Dir"=w334:path[])  [unwired: 4 in, 4 out]
            n158 = for {
              tunnel: w334 -> [w358] mode=indexing
              shift-right: [w372] -> w324
              shift-left: w350 -> [w382]
              shift-right: [w369] -> w344
              shift-left: w339 -> [w381]
              shift-right: [w368] -> w343
              shift-left: w349 -> [w377]
              shift-right: [w379] -> w328
              shift-left: w345 -> [w371]
              shift-right: [w370] -> w327
              shift-left: w345 -> [w380]
              tunnel: w348 -> [w375]
              shift-right: [w365] -> w326
              shift-left: w345 -> [w378]
              shift-right: [w367] -> w329
              shift-left: w345 -> [w376]
              tunnel: w342 -> [w374]
              shift-right: [w366] -> w331
              shift-left: w345 -> [w373]
              tunnel: w340 -> [w363]
              tunnel: w341 -> [w362]
              shift-right: [w359] -> w338
              shift-left: w333 -> [w360]
              w361 = T8[] [enum."sam", enum."ref"] items=["sam", "ref"]
              n159 = Strip Path(path=w358) -> (name=w357:string)  [unwired: 1 out]
              n160 = call "filename-manage.vi"("filename-action"=filename-action."getIDStock", "file name IN"=w357) -> ("string OUT"=w364:string)  [unwired: 7 in, 2 out]
              n161 = for {
                tunnel: w374 -> [w408]
                tunnel: w357 -> [w385]
                tunnel: w364 -> [w397]
                shift-right: [w406] -> w372
                shift-left: w382 -> [w417]
                shift-right: [w412] -> w379
                shift-left: w371 -> [w405]
                shift-right: [w404] -> w370
                shift-left: w380 -> [w413]
                shift-right: [w398] -> w365
                shift-left: w378 -> [w411]
                shift-right: [w399] -> w367
                shift-left: w376 -> [w409]
                shift-right: [w400] -> w366
                shift-left: w373 -> [w407]
                shift-right: [w401] -> w368
                shift-left: w377 -> [w410]
                shift-right: [w402] -> w369
                shift-left: w381 -> [w416]
                tunnel: w363 -> [w390]
                tunnel: w375 -> [w395]
                tunnel: w362 -> [w392]
                tunnel: w361 -> [w389] mode=indexing
                shift-right: [w386] -> w359
                shift-left: w360 -> [w387]
                tunnel: w358 -> [w384]
                # "internal key"
                n162 = Look In Map(map=w392, key=w389) -> (value=w391:string)  [unwired: 1 in, 1 out]
                n163 = Look In Map(map=w390, key=w389) -> (value=w388:i32)  [unwired: 1 in, 1 out]
                n164 = Concatenate Strings(w397, w391) -> (w396:string)
                n165 = Insert Into Map(map in=w395, key=3-lorentzian-parameters."side (S|R)", value=w388) -> (map out=w394:map{T2, dbl})  [unwired: 2 out]
                n166 = for {
                  shift-right: [w423] -> w403
                  shift-left: w394 -> [w424]
                  tunnel: w408 -> [w422] mode=indexing
                  tunnel: w385 -> [w420]
                  n167 = Unbundle(w422) -> ("key"=w421:T2, "filename-action"=w419:T18)
                  n168 = call "filename-manage.vi"("filename-action"=w419, "file name IN"=w420) -> ("number OUT"=w418:dbl)  [unwired: 7 in, 2 out]
                  n169 = Insert Into Map(map in=w424, key=w421, value=w418) -> (map out=w423:map{T2, dbl})  [unwired: 2 out]
                }
                n170 = in-place {
                  in-place-border: [w466] -> w415
                  in-place-border: w403 -> [w465]
                  n171 = in-place-map #2(w417, w396) -> (w464:map{T2, dbl}, w466:bool)  [unwired: 1 in]
                  n172 = for {
                    tunnel: w465 -> [w472] mode=indexing
                    shift-right: [w470] -> w463
                    shift-left: w464 -> [w471]
                    n173 = Unbundle(w472) -> ("key"=w469:T2, "number OUT"=w468:dbl)
                    n174 = Insert Into Map(map in=w471, key=w469, value=w468) -> (map out=w470:map{T2, dbl})  [unwired: 2 out]
                  }
                  n175 = in-place-map #2(w463, LVMapReplaceAction."Modify Entry only if found" ("action")) -> (w406:map{string, map{T2, dbl}})  [unwired: 2 out]
                }
                n176 = Not(x=w415) -> (.not. x?=w414:bool)
                n177 = case shown="True" w414 {
                  tunnel: w416 -> [w432 w462]
                  tunnel: [w432 w461] -> w402
                  tunnel: w385 -> [_ w460]
                  tunnel: w396 -> [_ w434]
                  tunnel: w413 -> [w430 w459]
                  tunnel: [w430 w458] -> w404
                  tunnel: w405 -> [w431 w457]
                  tunnel: [w431 w456] -> w412
                  tunnel: [w428 w455] -> w398
                  tunnel: w411 -> [w428 w454]
                  tunnel: w403 -> [_ w439]
                  tunnel: w410 -> [w429 w453]
                  tunnel: [w429 w452] -> w401
                  tunnel: [w427 w451] -> w399
                  tunnel: w409 -> [w427 w450]
                  tunnel: [w426 w441] -> w400
                  tunnel: w407 -> [w426 w440]
                  tunnel: w387 -> [w425 w436]
                  tunnel: [w425 w435] -> w386
                  tunnel: w384 -> [_ w433]
                  frame False {
                  }
                  frame True {
                    n178 = Look In Map(map=w439, key=3-lorentzian-parameters."set of (B|T)") -> (value=w442:dbl)  [unwired: 1 in, 1 out]
                    n179 = Look In Map(map=w439, key=3-lorentzian-parameters."side (S|R)") -> (value=w448:dbl)  [unwired: 1 in, 1 out]
                    n180 = Look In Map(map=w439, key=3-lorentzian-parameters."T (K)") -> (value=w446:dbl)  [unwired: 1 in, 1 out]
                    n181 = Look In Map(map=w439, key=3-lorentzian-parameters."B (T)") -> (value=w438:dbl)  [unwired: 1 in, 1 out]
                    n182 = Look In Map(map=w439, key=3-lorentzian-parameters."θ (deg)") -> (value=w437:dbl)  [unwired: 1 in, 1 out]
                    n183 = Insert Into Set(10:w442, 11:w440) -> (3:w441:set{dbl})  [unwired: 1 out]
                    n184 = Insert Into Set(10:w448, 11:w450) -> (3:w451:set{dbl})  [unwired: 1 out]
                    n185 = Insert Into Set(10:w446, 11:w454) -> (3:w455:set{dbl})  [unwired: 1 out]
                    n186 = Insert Into Set(10:w438, 11:w459) -> (3:w458:set{dbl})  [unwired: 1 out]
                    n187 = Insert Into Set(10:w437, 11:w457) -> (3:w456:set{dbl})  [unwired: 1 out]
                    n188 = Insert Into Map(map in=w453, key=w434, value=w439) -> (map out=w452:map{string, map{T2, dbl}})  [unwired: 2 out]
                    n189 = Insert Into Map(map in=w462, key=w434, value=w460) -> (map out=w461:map{string, string})  [unwired: 2 out]
                    n190 = Insert Into Map(map in=w436, key=w434, value=w433) -> (map out=w435:map{string, path})  [unwired: 2 out]
                  }
                }
              }
            }
            "all short filenames" <- w344
            "temps&degs" <- w343
            "mathematica thing" <- w324
            "all full filenames" <- w338
            n191 = local read "selector"() -> (w332:T10)
            n192 = in-place {
              in-place-border: w331 -> [w356]
              in-place-border: w329 -> [w355]
              in-place-border: w328 -> [w352]
              in-place-border: w327 -> [w353]
              in-place-border: w326 -> [w354]
              n193 = in-place-cluster #3(w332) -> ()  [unwired: 5 out]
              n194 = in-place-cluster #3("lookup.all set of"=w356, "lookup.all sides"=w355, "lookup.all T's"=w354, "lookup.all B's"=w353, "lookup.all θ's"=w352) -> (w330:T10)
            }
            n195 = local write "selector"(w330) -> ()
          }
          frame "action: update default values" {
            w477 = map{T2, cluster{"ζ":dbl, "ζ":dbl}[]} {}  # Size: 0
            (unwired) map{string, map{T2, dbl}} {} ("Map OUT")
            w475 = map{T2, dbl[]} {}  # Size: 0
            n196 = call "string parse mathematica list assosiated array -- V2.vi"("action"=3-lorentzian-heat-response_action."parse string" ("derivative"), "string IN"="default values string") -> ("Map OUT"=w478:map{string, map{T2, dbl}})  [unwired: 8 in, 1 out]
            n197 = for {
              tunnel: w478 -> [w504] mode=indexing
              tunnel: w473 -> [w503]
              shift-right: [w501] -> w476
              shift-left: w477 -> [w500]
              n198 = Unbundle(w504) -> ("Map"=w502:map{T2, dbl})  [unwired: 1 out]
              n199 = for {
                tunnel: w503 -> [w512] mode=indexing
                tunnel: w502 -> [w511]
                shift-right: [w506] -> w501
                shift-left: w500 -> [w505]
                # "parameter"
                # "temperatures"
                n200 = Look In Map(map=w511, key=w512) -> (value=w508:dbl)  [unwired: 1 in, 1 out]
                n201 = Look In Map(map=w505, key=w512) -> (value=w514:cluster{"ζ":dbl, "ζ":dbl}[])  [unwired: 1 in, 1 out]
                n202 = Look In Map(map=w511, key=3-lorentzian-parameters."T (K)" ("Plost: sweep window")) -> (value=w509:dbl)  [unwired: 1 in, 1 out]
                n203 = Bundle("ζ"=w509, "ζ"=w508) -> (w507:cluster{"ζ":dbl, "ζ":dbl})  [unwired: 1 in]
                n204 = Build Array (concatenate)(w514, w507) -> (w513:cluster{"ζ":dbl, "ζ":dbl}[])
                n205 = Insert Into Map(map in=w505, key=w512, value=w513) -> (map out=w506:map{T2, cluster{"ζ":dbl, "ζ":dbl}[]})  [unwired: 2 out]
              }
            }
            n206 = for {
              tunnel: w476 -> [w493] mode=indexing
              shift-right: [w490] -> w474
              shift-left: w475 -> [w489]
              # "sorted temperastures"
              # "parameter"
              # "temperastures"
              n207 = Unbundle(w493) -> ("Plost: sweep window"=w487:T2, w492:cluster{"ζ":dbl, "ζ":dbl}[])
              n208 = for {
                tunnel: w492 -> [w499] mode=indexing
                tunnel: [w498] -> w491 mode=indexing
                tunnel: [w497] -> w484 mode=indexing
                n209 = Unbundle(w499) -> ("ζ"=w498:dbl, "ζ"=w497:dbl)
              }
              n210 = call "array - sorted inexes.vi"("x"=w491) -> ("index array"=w483:i32[], "sorted array"=w485:dbl[])  [unwired: 9 in]
              n211 = Insert Into Map(map in=w489, key=3-lorentzian-parameters."T (K)", value=w485) -> (map out=w488:map{T2, dbl[]})  [unwired: 2 out]
              n212 = for {
                tunnel: w484 -> [w496]
                tunnel: w483 -> [w495] mode=indexing
                tunnel: [w494] -> w482 mode=indexing
                n213 = Index Array(array=w496, index=w495) -> (element=w494:dbl)
              }
              n214 = Insert Into Map(map in=w488, key=w487, value=w482) -> (map out=w490:map{T2, dbl[]})  [unwired: 2 out]
            }
            n215 = disable-structure shown="Disabled" {
              frame Disabled {
                # "2 3 4 0 1"
                # "2 3 4 5 6"
                # "5 6 2 3 4"
                n216 = call "array - sorted inexes.vi"() -> ()  [unwired: 10 in, 2 out]
              }
              frame Enabled {
              }
            }
            n217 = call "nanocal -- defaut parameter manager -- V1.vi"("action"=nanocal_--_defaut_parameter_manager_action--_V1."update", "internal map"=w474) -> ()  [unwired: 9 in, 1 out]
          }
          frame "action: empty string from filelist" {
            n218 = local read "file pattern"() -> (w516:string)
            n219 = local read "folder"() -> (w517:path)
            n220 = call <vilib>:"Recursive File List.vi"("pattern"=w516, "Continue Recursing on Error? (F)"=TRUE, "Folder Path"=w517) -> ("All Files in Dir"=w515:path[])  [unwired: 4 in, 4 out]
            n221 = for {
              tunnel: [w522] -> w519 mode=concatenating
              tunnel: w515 -> [w527] mode=indexing
              w525 = T8[] [enum."ref", enum."sam"] items=["sam", "ref"]
              n222 = Strip Path(path=w527) -> (name=w526:string)  [unwired: 1 out]
              n223 = local read "side map to STR"() -> (w524:map{T8, string})
              n224 = call "filename-manage.vi"("filename-action"=filename-action."getIDStock", "file name IN"=w526) -> ("string OUT"=w523:string)  [unwired: 7 in, 2 out]
